vi "ScanImage.vi"(11 "Scan Info":T1={"X Center"=0.0, "Y Center"=0.0, "Width"=1.0, "Height"=1.0, "Time [ms]"=1000.0, "As Dwell Time"=FALSE, "Pixels"=300.0}) -> ()   [LabVIEW 2017]
uses:
  Types/ScanInfo.ctl
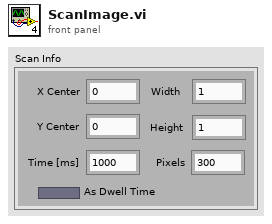
[diagram p1: front panel]
types:
  T1 = typedef "ScanInfo.ctl" = cluster{"X Center":dbl, "Y Center":dbl, "Width":dbl, "Height":dbl, "Time [ms]":dbl, "As Dwell Time":bool, "Pixels":dbl}
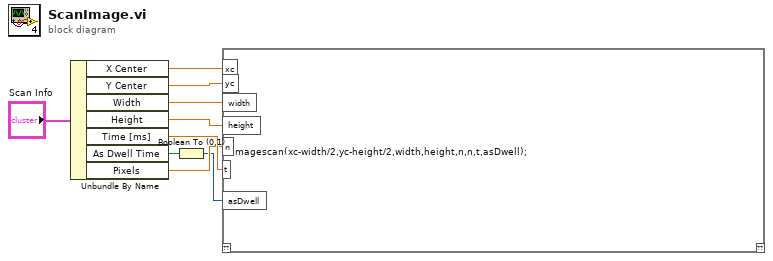
[diagram p0: block diagram]
diagram:
  n1 = Unbundle By Name("Scan Info") -> ("X Center"=w4:dbl, "Y Center"=w3:dbl, "Width"=w6:dbl, "Height"=w5:dbl, "Time [ms]"=w8:dbl, "As Dwell Time"=w2:bool, "Pixels"=w7:dbl)
  n2 = Boolean To (0,1)(Boolean=w2) -> (0, 1=w1:i16)
  n3 = script code="imagescan(xc-width/2,yc-height/2,width,height,n,n,t,asDwell);"("xc"=w4, "yc"=w3, "width"=w6, "height"=w5, "n"=w7, "t"=w8, "asDwell"=w1) -> ()  [unwired: 1 in, 1 out]
